vi "CreateParseBody.vi"(8 "error in (no error)":errorcluster, 10 "Message in":T1, 11 "VI reference":refnum<vi>) -> (0 "error out":errorcluster)   [LabVIEW 2017, in "MessageGen.lvlib"]
uses:
  <vilib>/addons/InsightCM/MessageBus/CodeGen/MessageGen.lvlib
  <vilib>/addons/InsightCM/MessageBus/CodeGen/controls/MessageData.ctl
  <vilib>/addons/InsightCM/MessageBus/CodeGen/controls/MessageType.ctl
  <vilib>/addons/InsightCM/MessageBus/CodeGen/controls/Parameter.ctl
  <vilib>/addons/InsightCM/MessageBus/CodeGen/controls/ParameterType.ctl
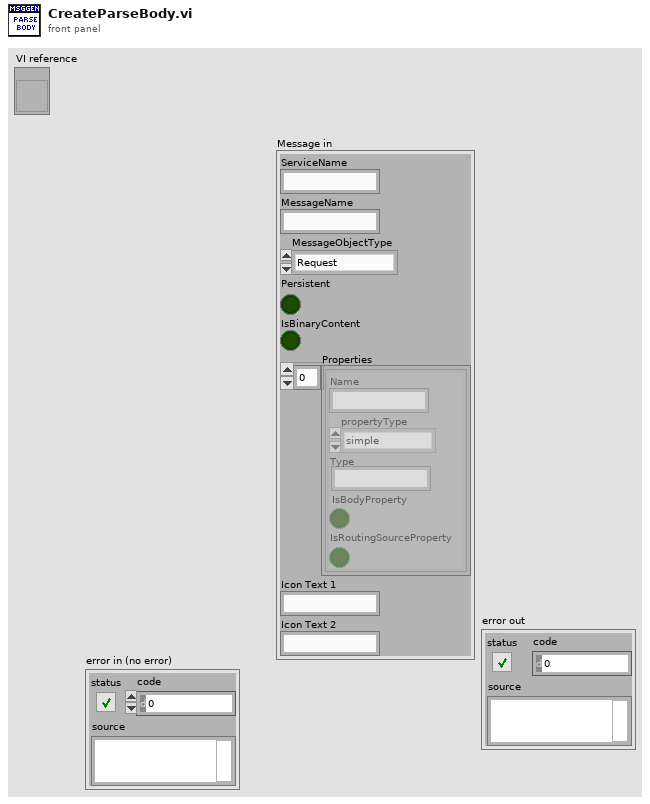
[diagram p1: front panel]
types:
  T1 = typedef "MessageGen.lvlib/MessageData.ctl" = cluster{"ServiceName":string, "MessageName":string, "MessageObjectType":T2, "Persistent":bool, "IsBinaryContent":bool, "Properties":T3[], "Icon Text 1":string, "Icon Text 2":string}
  T2 = typedef "MessageGen.lvlib/MessageType.ctl" = enum16{"Request", "Response", "Broadcast", "RoutedMessage"}
  T3 = typedef "MessageGen.lvlib/Parameter.ctl" = cluster{"Name":string, "propertyType":T4, "Type":string, "IsBodyProperty":bool, "IsRoutingSourceProperty":bool}
  T4 = typedef "MessageGen.lvlib/ParameterType.ctl" = enum16{"simple", "bytearray", "dateTime", "list", "map", "object"}
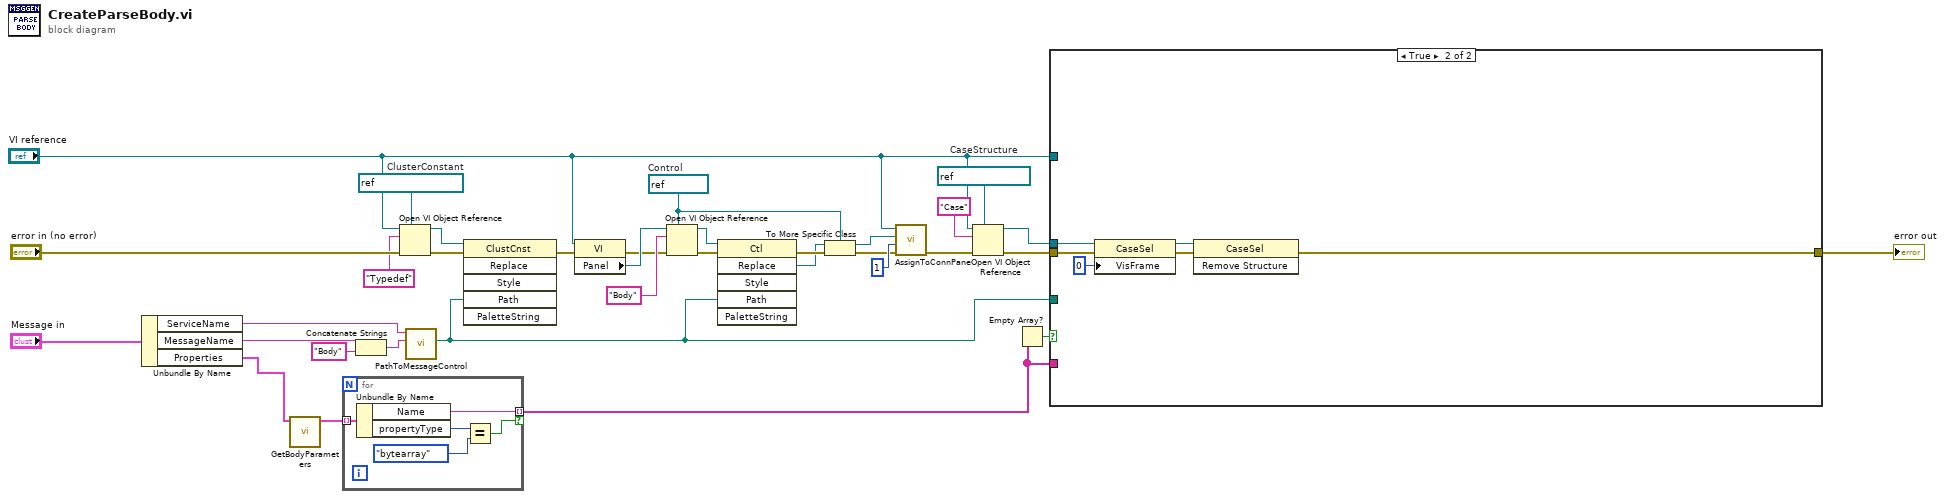
[diagram p0: block diagram]
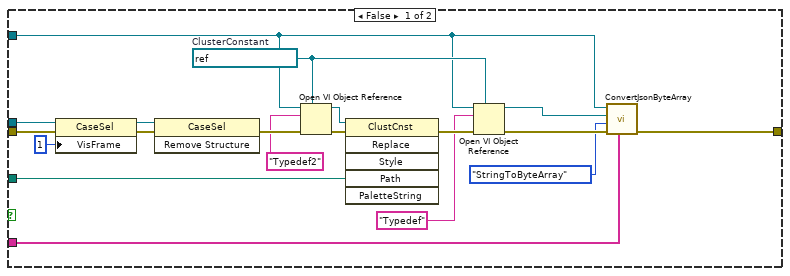
[diagram p2: hidden frame]
diagram:
  w2 = refnum<vi> refnum  # Control
  w16 = refnum<vi> refnum  # ClusterConstant
  w25 = refnum<vi> refnum  # CaseStructure
  n1 = Unbundle By Name("Message in") -> ("ServiceName"=w31:string, "MessageName"=w30:string, "Properties"=w33:T3[])
  n2 = call <vilib>:"GetBodyParameters.vi"("Parameters"=w33) -> ("BodyParameters"=w23:T3[])  [unwired: 9 in, 1 out]
  n3 = for {
    tunnel: w23 -> [w39] mode=indexing
    tunnel: [w37] -> w22 mode=indexing if=w35
    n4 = Unbundle By Name(w39) -> ("Name"=w37:string, "propertyType"=w38:T4)
    n5 = Equal?(x=w38, y=ParameterType."bytearray" ("x")) -> (x = y?=w35:bool)
  }
  n6 = Concatenate Strings(w30, "Body" ("string")) -> (w21:string)
  n7 = Open VI Object Reference(7:w16, 8:"error in (no error)", 10:"Typedef" ("name/order"), 11:"VI reference") -> (0:w17:errorcluster, 3:w18:refnum<vi>)
  n8 = call <vilib>:"PathToMessageControl.vi"("ControlName"=w21, "Service"=w31) -> ("Path"=w8:path)  [unwired: 9 in]
  n9 = invoke class="ClustCnst" method="Replace"(reference=w18, error in=w17, "Path"=w8) -> (error out=w9:errorcluster)  [unwired: 3 in, 5 out]
  n10 = property class="VI"(reference="VI reference", error in=w9) -> (error out=w12:errorcluster, "Panel"=w13:refnum<vi>)  [unwired: 1 out]
  n11 = Open VI Object Reference(7:w2, 8:w12, 10:"Body" ("name/order"), 11:w13) -> (0:w10:errorcluster, 3:w11:refnum<vi>)
  n12 = invoke class="Ctl" method="Replace"(reference=w11, error in=w10, "Path"=w8) -> (error out=w5:errorcluster, "Replace"=w3:refnum<vi>)  [unwired: 3 in, 4 out]
  n13 = To More Specific Class(target class=w2, reference=w3, error in=w5) -> (specific class reference=w1:refnum<vi>, error out=w4:errorcluster)
  n14 = call <vilib>:"AssignToConnPane.vi"("error in (no error)"=w4, "term index"=u32 1, "Control"=w1, "vi reference"="VI reference") -> ("error out"=w7:errorcluster)  [unwired: 7 in]
  n15 = Open VI Object Reference(7:w25, 8:w7, 10:"Case" ("name/order"), 11:"VI reference") -> (0:w27:errorcluster, 3:w28:refnum<vi>)
  n16 = Empty Array?(array=w22) -> (empty?=w26:bool)
  n17 = case shown="True" w26 {
    tunnel: [w40 w59] -> w29
    tunnel: "VI reference" -> [w48 _]
    tunnel: w27 -> [w50 w61]
    tunnel: w28 -> [w49 w60]
    tunnel: w22 -> [w43 _]
    tunnel: w8 -> [w41 _]
    frame False {
      w55 = refnum<vi> refnum  # ClusterConstant
      n18 = property class="CaseSel"(reference=w49, error in=w50, "VisFrame"=u32 1 ("Visible Frame")) -> (reference out=w52:refnum<vi>, error out=w53:errorcluster)
      n19 = invoke class="CaseSel" method="Remove Structure"(reference=w52, error in=w53) -> (error out=w54:errorcluster)  [unwired: 1 in, 2 out]
      n20 = Open VI Object Reference(7:w55, 8:w54, 10:"Typedef2" ("name/order"), 11:w48) -> (0:w57:errorcluster, 3:w56:refnum<vi>)
      n21 = invoke class="ClustCnst" method="Replace"(reference=w56, error in=w57, "Path"=w41) -> (error out=w58:errorcluster)  [unwired: 3 in, 5 out]
      n22 = Open VI Object Reference(7:w55, 8:w58, 10:"Typedef" ("name/order"), 11:w48) -> (0:w44:errorcluster, 3:w45:refnum<vi>)
      n23 = call <vilib>:"ConvertJsonByteArray.vi"("controls to convert"=w43, "error in (no error)"=w44, "direction"=enum16{"ByteArrayToString", "StringToByteArray"}."StringToByteArray", "cluster to disconnect"=w45, "VI ref"=w48) -> ("error out"=w40:errorcluster)  [unwired: 6 in]
    }
    frame True {
      n24 = property class="CaseSel"(reference=w60, error in=w61, "VisFrame"=u32 0 ("Visible Frame")) -> (reference out=w63:refnum<vi>, error out=w64:errorcluster)
      n25 = invoke class="CaseSel" method="Remove Structure"(reference=w63, error in=w64) -> (error out=w59:errorcluster)  [unwired: 1 in, 2 out]
    }
  }
  "error out" <- w29
